vi "Start.vi"(5 "Cluster":string, 6 "Bind Address":string, 7 "System":string, 8 "error in (no error)":errorcluster, 9 "DiscoveryPort":u16, 10 "Discovery Address":string, 11 "TelemetryDebug in":refnum<class "TelemetryDebug.lvclass">) -> (0 "error out":errorcluster, 3 "TelemetryDebug out":refnum<class "TelemetryDebug.lvclass">)   [LabVIEW 2020, in "VectoTools.lvlib" / "TelemetryDebug.lvclass"]
uses:
  TelemetryDebug.lvclass
  Vecto/Node Config/Node Info.ctl
  Vecto/Node Config/Discovery Info.ctl
  Vecto/EventLoggingService/EventLoggingService.lvclass
  TelemetryDebug.lvclass/TelemetryDebug.ctl
  Vecto/DiscoveryService/DiscoveryService.lvclass
  Vecto/Node Config/Node Config.lvclass
  VectoConfig/VectoConfig.lvlib
  Vecto/SequenceCountService/SequenceCountService.lvclass
  Vecto/RemoteDataService/RemoteDataService.lvclass
  Vecto/ChannelService/ChannelService.lvclass
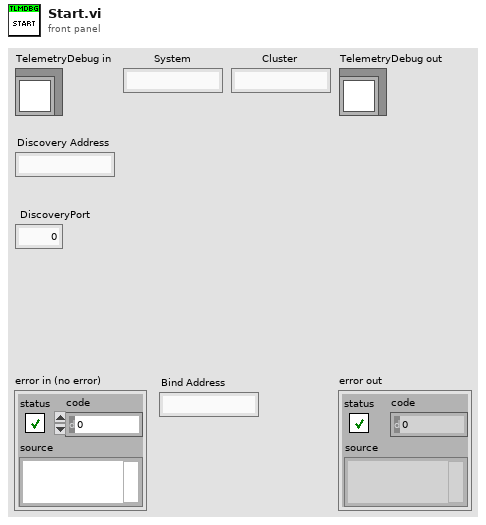
[diagram p1: front panel]
types:
  T1 = typedef "VectoConfig.lvlib/Discovery Info.ctl" = cluster{"Address":string, "Port":u16, "Interval S":dbl, "Bind Address":string}
  T2 = typedef "VectoConfig.lvlib/Node Info.ctl" = cluster{"System":string, "Cluster":string, "Name":string, "ID":u32, "Capabilities":string[]}
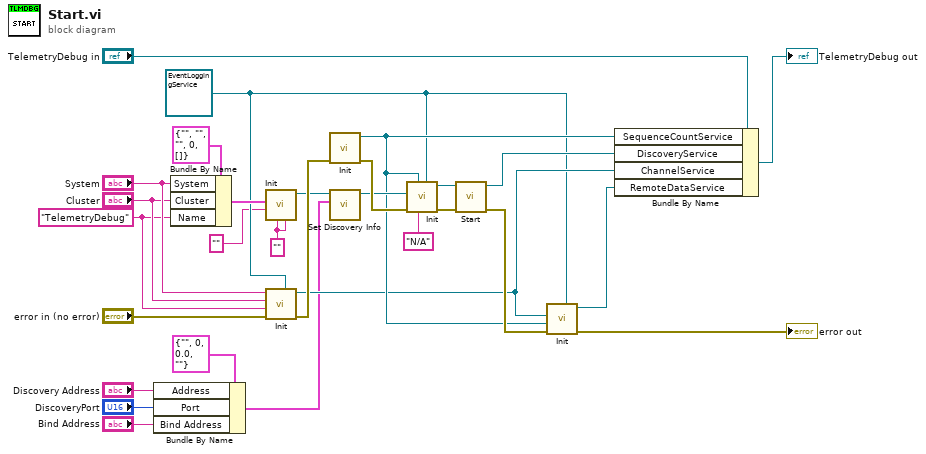
[diagram p0: block diagram]
diagram:
  w2 = "" ("Config Version")
  w3 = refnum<class "EventLoggingService.lvclass"> refnum ("Vecto.lvlib:EventLoggingService.lvclass")
  w13 = "TelemetryDebug" ("Name")
  n1 = Bundle By Name(cluster=T1 {"Address"="", "Port"=0, "Interval S"=0.0, "Bind Address"=""} ("Discovery Info"), "Address"="Discovery Address", "Port"="DiscoveryPort", "Bind Address"="Bind Address") -> (w6:T1)
  n2 = Bundle By Name(cluster=T2 {"System"="", "Cluster"="", "Name"="", "ID"=0, "Capabilities"=[]} ("Node Info"), "System"="System", "Cluster"="Cluster", "Name"=w13) -> (w25:T2)
  n3 = call "Init.vi"("Config Hash"=w2, "Config Version"=w2, "Alias (None)"="", "Node Info"=w25) -> ("Node out"=w24:refnum<class "Node Config.lvclass">)  [unwired: 6 in, 1 out]
  n4 = call "Init.vi"("EventLogger"=w3, "error in (no error)"="error in (no error)", "Node"=w13, "Cluster"="Cluster", "System"="System") -> ("error out"=w29:errorcluster, "ChannelService out"=w12:refnum<class "ChannelService.lvclass">)  [unwired: 5 in]
  n5 = call "Init.vi"("error in (no error)"=w29) -> ("error out"=w27:errorcluster, "SequenceCountService out"=w16:refnum<class "SequenceCountService.lvclass">)  [unwired: 9 in]
  n6 = call "Set Discovery Info.vi"("Discovery Info"=w6, "Node in"=w24) -> ("Node out"=w22:refnum<class "Node Config.lvclass">)  [unwired: 8 in, 1 out]
  n7 = call "Init.vi"("EventLogger"=w3, "App Version"="N/A", "SequenceCountService"=w16, "error in (no error)"=w27, "Node"=w22) -> ("error out"=w20:errorcluster, "DiscoveryService out"=w21:refnum<class "DiscoveryService.lvclass">)  [unwired: 5 in]
  n8 = call "Start.vi"("error in (no error)"=w20, "DiscoveryService in"=w21) -> ("error out"=w28:errorcluster, "DiscoveryService out"=w17:refnum<class "DiscoveryService.lvclass">)  [unwired: 8 in]
  n9 = call "Init.vi"("EventLogger"=w3, "error in (no error)"=w28, "SequenceCountService"=w16, "ChannelService"=w12) -> ("error out"=→"error out":errorcluster, "RemoteDataService out"=w11:refnum<class "RemoteDataService.lvclass">)  [unwired: 6 in]
  n10 = Bundle By Name(cluster="TelemetryDebug in", "SequenceCountService"=w16, "DiscoveryService"=w17, "ChannelService"=w12, "RemoteDataService"=w11) -> (→"TelemetryDebug out":refnum<class "TelemetryDebug.lvclass">)
